vi "PCU_Get_Power_Range.vi"(8 "error in (no error)":errorcluster, 11 ".NET Reference in":refnum<k24>) -> (0 "error out":errorcluster, 2 "range":i32, 3 "Reference out":refnum<k24>)   [LabVIEW 2017]
uses:
  C:/Users/Ssantec_Test/Documents/Instrument_DLL_Sample_Labview_20220902_Ver1.2.2/DLL/x86/InstrumentDLL.dll
  DLL/x86/InstrumentDLL.dll
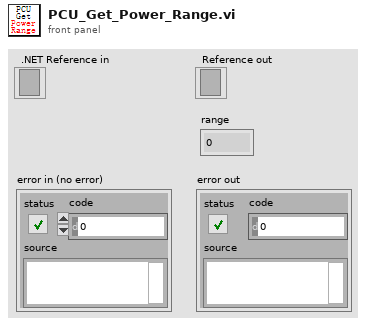
[diagram p1: front panel]
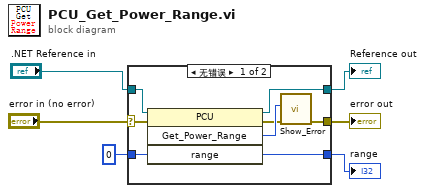
[diagram p0: block diagram]
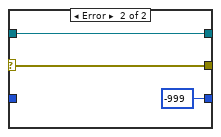
[diagram p2: hidden frame]
diagram:
  n1 = case shown="无错误" "error in (no error)" {
    selector: "error in (no error)" -> [w10 w17]
    tunnel: [w14 -999 ("range")] -> w6
    tunnel: 0 ("range") -> [w13 _]
    tunnel: ".NET Reference in" -> [w12 w16]
    tunnel: [w11 w16] -> w3
    tunnel: [w7 w17] -> w2
    frame No Error {
      n2 = invoke on="调用节点" class="PCU" method="Get_Power_Range"(reference=w12, error in=w10, "range"=w13) -> (reference out=w11:refnum<k24>, error out=w8:errorcluster, "Get_Power_Range"=w9:i32, "range"=w14:i32)  [unwired: 1 in]
      n3 = call "Show_Error.vi"("error in (no error)"=w8, "Error"=w9) -> ("error out"=w7:errorcluster)  [unwired: 9 in]
    }
    frame Error {
    }
  }
  "range" <- w6
  "Reference out" <- w3
  "error out" <- w2
